vi "Write Lower Limit.vi"(8 "error in (no error)":errorcluster, 10 "Lower Limit":dbl, 11 "Test Double Float in":refnum<class "Test Double Float.lvclass">) -> (0 "error out":errorcluster, 3 "Test Double Float out":refnum<class "Test Double Float.lvclass">)   [LabVIEW 2021, in "BT.lvlib" / "Test Double Float.lvclass"]
uses:
  Test Double Float.lvclass
  Test Double Float.lvclass/Test Double Float.ctl
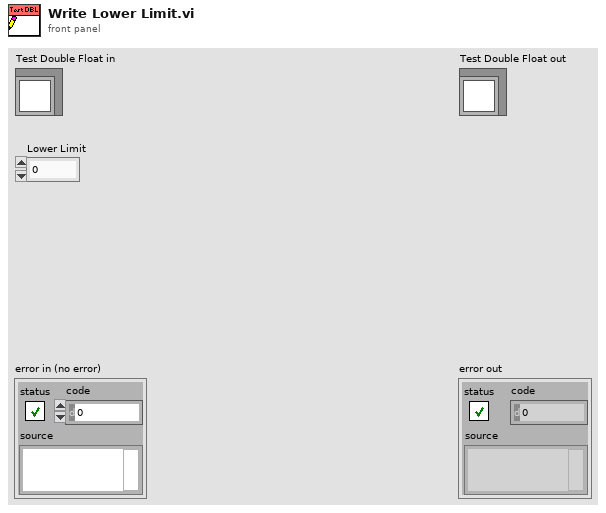
[diagram p1: front panel]
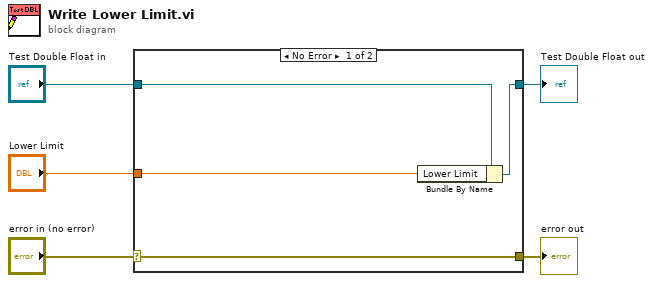
[diagram p0: block diagram]
diagram:
  n1 = case shown="No Error" "error in (no error)" {
    selector: "error in (no error)" -> [w9 w10]
    tunnel: [w9 w10] -> w4
    tunnel: [w7 w11] -> w2
    tunnel: "Test Double Float in" -> [w8 w11]
    tunnel: "Lower Limit" -> [w6 _]
    frame No Error {
      n2 = Bundle By Name(cluster=w8, "Lower Limit"=w6) -> (w7:refnum<class "Test Double Float.lvclass">)
    }
    frame Error {
    }
  }
  "error out" <- w4
  "Test Double Float out" <- w2
